vi "Connect.vi"(8 "error in (no error)":errorcluster, 11 "TCP_Client in":refnum<class "TCP_Client.lvclass">) -> (0 "error out":errorcluster, 3 "TCP_Client out":refnum<class "TCP_Client.lvclass">)   [LabVIEW 2018, in "TCP_Client.lvlib" / "TCP_Client.lvclass"]
uses:
  TCP_Client.lvclass
  TCP_Client.lvclass/TCP_Client.ctl
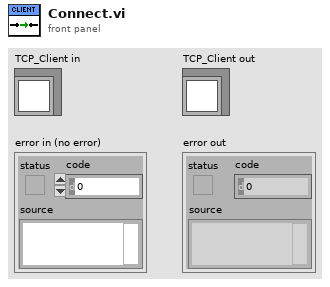
[diagram p1: front panel]
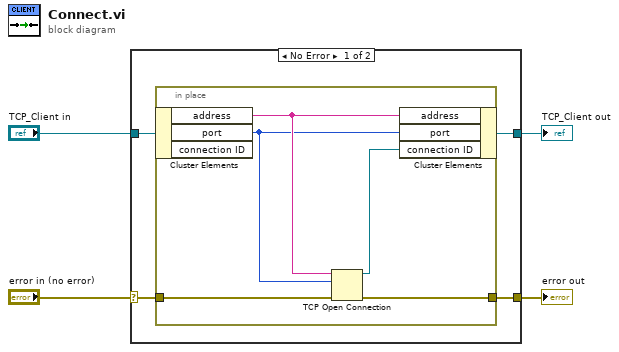
[diagram p0: block diagram]
diagram:
  n1 = case shown="No Error" "error in (no error)" {
    selector: "error in (no error)" -> [w8 w15]
    tunnel: [w5 w15] -> w3
    tunnel: [w6 w14] -> w1
    tunnel: "TCP_Client in" -> [w7 w14]
    frame No Error {
      n2 = in-place {
        in-place-border: w8 -> [w13]
        in-place-border: [w11] -> w5
        n3 = in-place-cluster #1(w7) -> ("address"=w10:string, "port"=w9:u16)  [unwired: 1 out]
        n4 = TCP Open Connection(address=w10, remote port or service name=w9, error in (no error)=w13) -> (connection ID=w12:refnum<k5>, error out=w11:errorcluster)  [unwired: 2 in]
        n5 = in-place-cluster #1("address"=w10, "port"=w9, "connection ID"=w12) -> (w6:refnum<class "TCP_Client.lvclass">)
      }
    }
    frame Error {
    }
  }
  "error out" <- w3
  "TCP_Client out" <- w1
